vi "PROJECTE OCELL versió 0.2.vi"() -> ()   [LabVIEW 2020]
uses:
  <vilib>/MakerHub/LINX/Public/Utilities/Open Serial.vi
  <vilib>/MakerHub/LINX/LMH-LINX.lvlib
  <vilib>/MakerHub/LINX/Public/Sensors/Distance/Ultrasonic/Ultrasonic.lvlib
panel:
  in  "sensibilitat 2":i64
  in  "sensibilitat 1":i64
  out "Error Out 2":errorcluster
  out "Centimeters":dbl(slide) scale=0.0..50.0
  in  "DO Channel 2":u8
  in  "DI Channel   2":u8
  out "Centímetres":dbl(slide) scale=0.0..50.0
  in  "DO Channel":u8
  out "appended array":cluster{i32[], dbl[]}[](array[cluster])
  in  "Velocitat de moviment":u32=100
  out "Error Out":errorcluster
  in  "DI Channel":u8
  out "Device Name":string
  in  "Error In":errorcluster
  in  "Baud Rate Override":u32=9600
  in  "Serial Port":refnum<visa-resource-name>="N/A"
  out "Monitor":cluster{i32[], i64[]}[](graph)
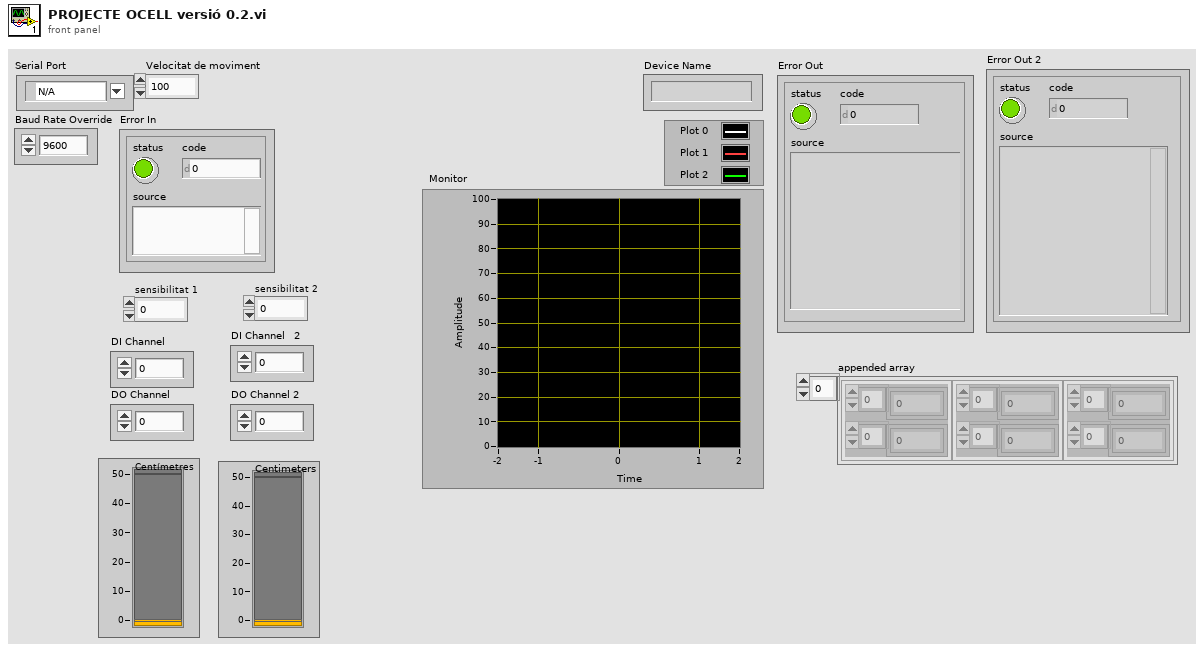
[diagram p1: front panel]
types:
  T1 = typedef "LMH-LINX.lvlib/LINX Ref.ctl" = cluster{"IO":T2, "Interface":T3, "LINX Device Config":T4}
  T2 = typedef "LMH-LINX.lvlib/Platform.ctl" = enum16{"Remote", "Local"}
  T3 = typedef "LMH-LINX.lvlib/Interface.ctl" = enum16{"Serial", "TCP"}
  T4 = typedef "LMH-LINX.lvlib/Device.lvlib/LINX Device Config.ctl" = cluster{"Interface":T3, "COM Port":refnum<visa-resource-name>, "TCP Configuration":T5, "Device Family":u8, "Device ID":u8, "Device Name":string, "TCP Ref":refnum<k5>, "Channels":T6}
  T5 = typedef "LMH-LINX.lvlib/Device.lvlib/TCP Config.ctl" = cluster{"IP Address":string, "Port":u16}
  T6 = typedef "LMH-LINX.lvlib/Channels.ctl" = cluster{"DI":u8[], "DO":u8[], "AI":u8[], "AO":u8[], "PWM":u8[], "QE":u8[], "UART":u8[], "I2C 2":u8[], "SPI":u8[], "CAN":u8[], "Servo":u8[], "AI Ref (V)":dbl, "AI Resolution (Bits)":u8, "AO Ref (V)":dbl, "AO Resolution (Bits)":u8}
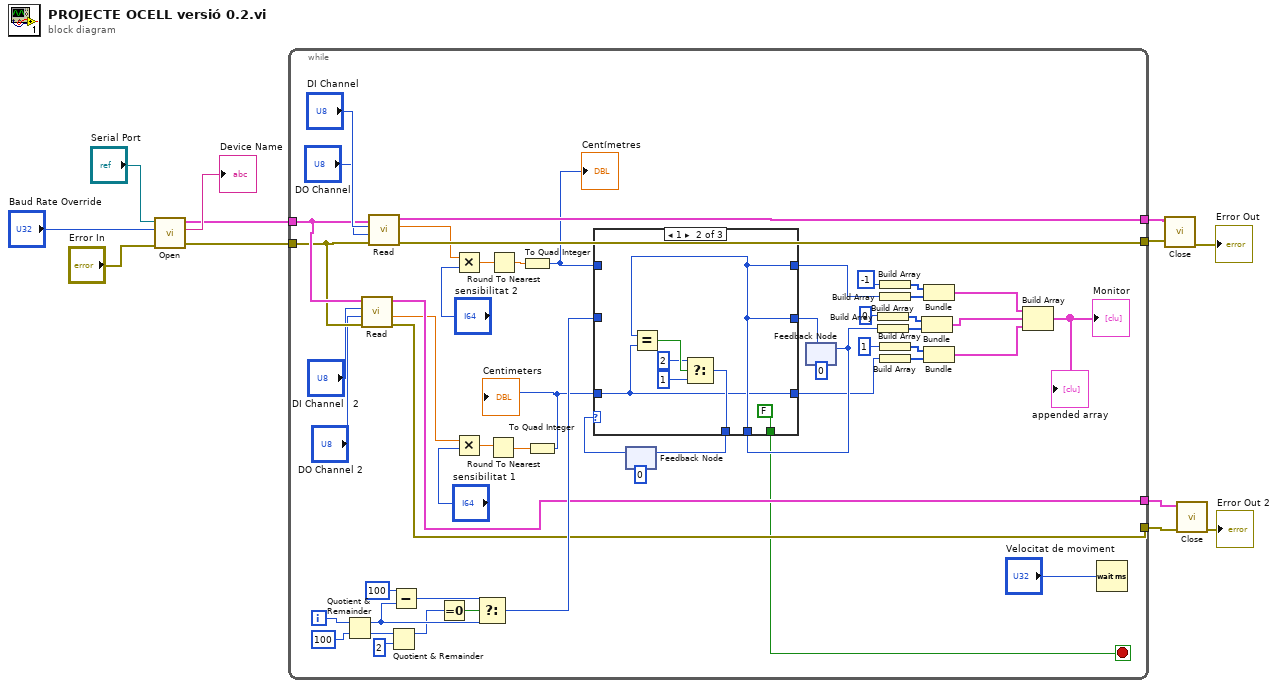
[diagram p0: block diagram]
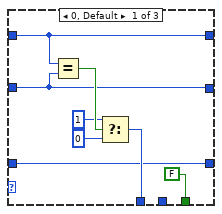
[diagram p2: hidden frame]
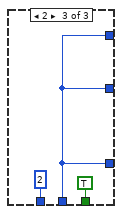
[diagram p3: hidden frame]
diagram:
  n1 = call-poly <vilib>:"Open.vi"("Error In"="Error In", "Baud Rate Override"="Baud Rate Override", "Serial Port"="Serial Port") -> ("Error Out"=w8:errorcluster, "Device Name"=→"Device Name":string, "LINX Resource"=w9:T1)  [unwired: 6 in]
  n2 = while {
    tunnel: w9 -> [w30]
    tunnel: w8 -> [w29]
    tunnel: [w26] -> w7
    tunnel: [w60] -> w6
    tunnel: [w24] -> w3
    tunnel: [w25] -> w2
    i -> [w50]
    stop <- w13 stop-if-true
    n3 = Quotient & Remainder(x=w50, y=100) -> (x-y*floor(x/y)=w47:i32, floor(x/y)=w44:i32)
    n4 = call <vilib>:"Read.vi"("Error In"=w29, "DO Channel"="DO Channel 2", "DI Channel"="DI Channel   2", "LINX Resource"=w30) -> ("Error Out"=w25:errorcluster, "Centimeters"=w17:dbl, "LINX Resource"=w24:T1)  [unwired: 4 in, 1 out]
    n5 = call <vilib>:"Read.vi"("Error In"=w29, "DO Channel"="DO Channel", "DI Channel"="DI Channel", "LINX Resource"=w30) -> ("Error Out"=w60:errorcluster, "Inches"=w20:dbl, "LINX Resource"=w26:T1)  [unwired: 4 in, 1 out]
    n6 = Quotient & Remainder(x=w44, y=2) -> (x-y*floor(x/y)=w42:i32)  [unwired: 1 out]
    n7 = Subtract(x=100 ("y"), y=w47) -> (x-y=w46:i32)
    n8 = Equal To 0?(x=w42) -> (x = 0?=w43:bool)
    n9 = Multiply(x=w20, y="sensibilitat 2") -> (x*y=w19:dbl)
    n10 = Multiply(x=w17, y="sensibilitat 1") -> (x*y=w15:dbl)
    n11 = Select(t=w46, s=w43, f=w47) -> (s? t:f=w39:i32)
    n12 = Round To Nearest(number=w15) -> (nearest integer value=w16:dbl)
    n13 = Round To Nearest(number=w19) -> (nearest integer value=w21:dbl)
    n14 = To Quad Integer(1:w21) -> (0:w18:i64)
    "Centímetres" <- w18
    n15 = To Quad Integer(1:w16) -> (0:w14:i64)
    "Centimeters" <- w14
    n16 = feedback #1(0 ("f")) -> (w33:i32)
    n17 = feedback #2(0) -> (w37:i32)
    n18 = case shown="1" w33 {
      tunnel: w18 -> [w73 _ _]
      tunnel: [w73 w76 w82] -> w41
      tunnel: w39 -> [w70 _ _]
      tunnel: [w70 w76 w82] -> w38
      tunnel: w37 -> [_ w76 w82]
      tunnel: w14 -> [w68 w75 _]
      tunnel: [w68 w75 w82] -> w35
      tunnel: [w71 w77 2 ("f")] -> w34
      tunnel: [FALSE FALSE TRUE] -> w13
      frame 0, Default {
        n19 = Equal?(x=w73, y=w70) -> (x = y?=w72:bool)
        n20 = Select(t=1, s=w72, f=0) -> (s? t:f=w71:i32)
      }
      frame 1 {
        n21 = Equal?(x=w76, y=w75) -> (x = y?=w80:bool)
        n22 = Select(t=2, s=w80, f=1) -> (s? t:f=w77:i32)
      }
      frame 2 {
      }
    }
    n23 = feedback-in #1(w34) -> ()
    n24 = feedback-in #2(w38) -> ()
    n25 = Build Array(0) -> (w54:i32[])
    n26 = Build Array(w37) -> (w40:i32[])
    n27 = Build Array(-1) -> (w56:i32[])
    n28 = Build Array(w41) -> (w57:i64[])
    n29 = Build Array(1) -> (w52:i32[])
    n30 = Build Array(w35) -> (w51:i64[])
    n31 = Bundle(w54, w40) -> (w63:cluster{i32[], i32[]})  [unwired: 1 in]
    n32 = Bundle(w56, w57) -> (w64:cluster{i32[], i64[]})  [unwired: 1 in]
    n33 = Bundle(w52, w51) -> (w62:cluster{i32[], i64[]})  [unwired: 1 in]
    n34 = Build Array(w64, w63, w62) -> (→"Monitor" →"appended array":cluster{i32[], i64[]}[])
    n35 = Wait (ms)(milliseconds to wait="Velocitat de moviment") -> ()  [unwired: 1 out]
  }
  n36 = call <vilib>:"Close.vi"("Error In"=w6, "LINX Resource"=w7) -> ("Error Out"=→"Error Out":errorcluster)  [unwired: 9 in]
  n37 = call <vilib>:"Close.vi"("Error In"=w2, "LINX Resource"=w3) -> ("Error Out"=→"Error Out 2":errorcluster)  [unwired: 9 in]
